vi "Biosignal program_190528.vi"() -> ()   [LabVIEW 2013]
uses:
  <vilib>/express/express analysis/Spectral/Block/exnSpectralBlock spectral measurements power poly.vi
  <vilib>/express/express analysis/Spectral/Block/exnSpectralBlock spectral measurements power DDT.vi
  <vilib>/express/express analysis/Spectral/XNode/ExpressSpectralMeasurementsBlockNode.xnode
panel:
  out "Numeric":dbl
  in  "Reset":bool
  out "Bandpassed signal":dynamicdata(graph)
  in  "Lowpass Freq.":dbl
  in  "Highpass Freq.":dbl
  in  "Samples to read":dbl
  in  "Sampling freq":dbl
  in  "Write to text":bool
  in  "stop":bool
  in  "File name":path
  out "DATA":dynamicdata(graph)
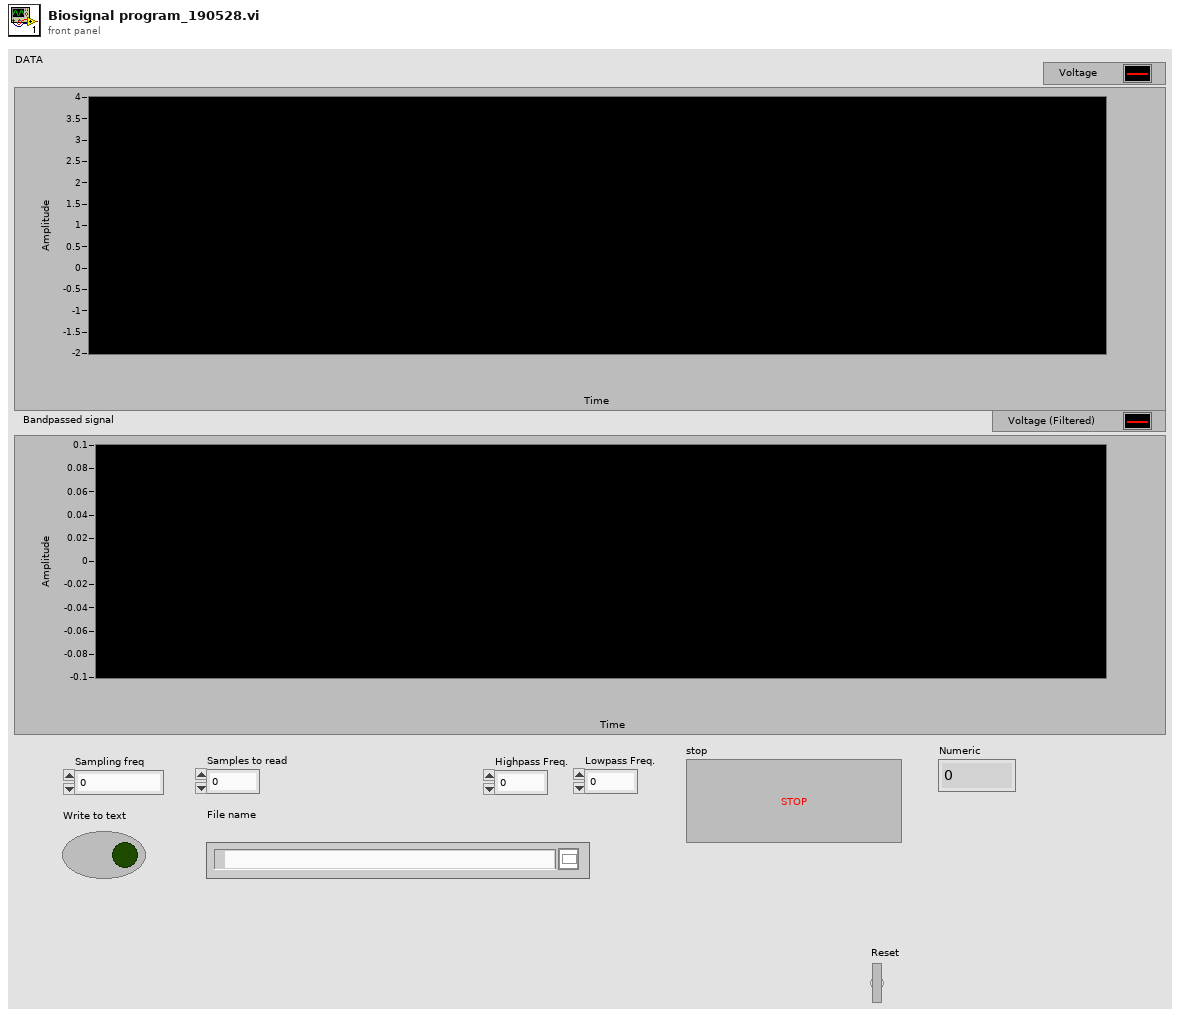
[diagram p1: front panel]
types:
  T1 = cluster{"averaging mode":u16, "weighting mode":u16, "number of averages":u32}
  T2 = cluster{"dB On (F)":bool, "unwrap phase (F)":bool, "convert to degree (F)":bool}
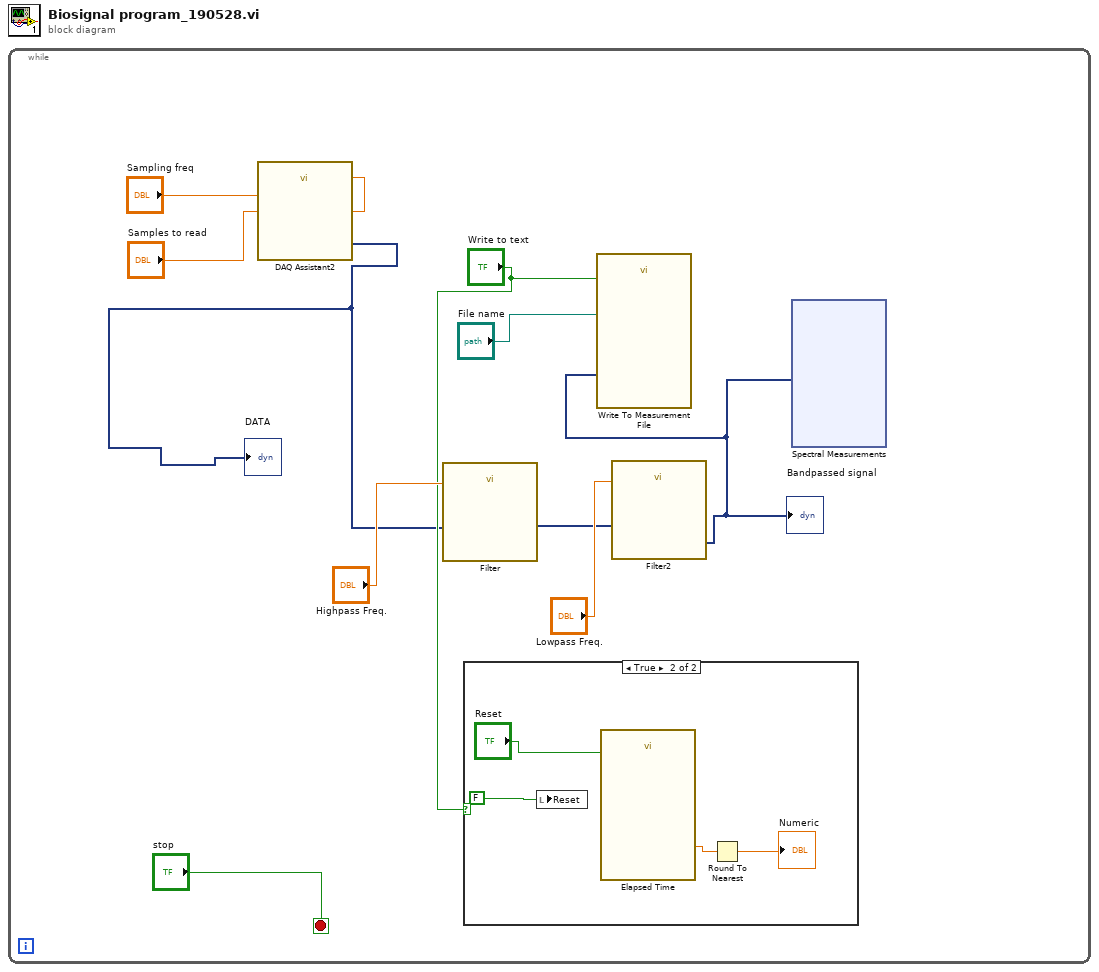
[diagram p0: block diagram]
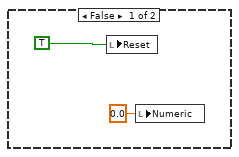
[diagram p2: hidden frame]
diagram:
  n1 = while {
    stop <- "stop" stop-if-true
    n2 = call "DAQ Assistant2"("rate"="Sampling freq", "number of samples"="Samples to read") -> ("data"=w4:dynamicdata)  [unwired: 14 in, 3 out]
    "DATA" <- w4
    n3 = call "Filter"("Lower Cut-Off"="Highpass Freq.", "Signal"=w4) -> ("Filtered Signal"=w5:dynamicdata)  [unwired: 8 in, 1 out]
    n4 = case shown="True" "Write to text" {
      frame False {
        n5 = local write "Reset"(TRUE) -> ()
        n6 = local write "Numeric"(0.0 ("Numeric")) -> ()
      }
      frame True {
        n7 = local write "Reset"(FALSE) -> ()
        n8 = call "Elapsed Time"("Reset"="Reset") -> ("Elapsed Time (s)"=w16:dbl)  [unwired: 11 in, 7 out]
        n9 = Round To Nearest(number=w16) -> (nearest integer value=→"Numeric":dbl)
      }
    }
    n10 = call "Filter2"("Lower Cut-Off"="Lowpass Freq.", "Signal"=w5) -> ("Filtered Signal"=w1:dynamicdata)  [unwired: 8 in, 1 out]
    "Bandpassed signal" <- w1
    n11 = call "Write To Measurement File"("Signals"=w1, "Enable"="Write to text", "Filename"="File name") -> ()  [unwired: 14 in, 3 out]
    n12 = xnode "Spectral Measurements"("Signals"=w1) -> ()  [unwired: 1 in, 2 out]
  }
